vi "Read TopicLookupTable.vi"(11 "Mediator in":refnum<class "Mediator.lvclass">) -> (2 "TopicLookupTable":refnum<data-value>)   [LabVIEW 2018, in "MVA Framework.lvlib" / "Mediator.lvlib" / "Mediator.lvclass"]
doc: "读取主题查找表"
uses:
  Mediator.lvclass
  TopicLookupTable/TopicLookupTable.lvclass
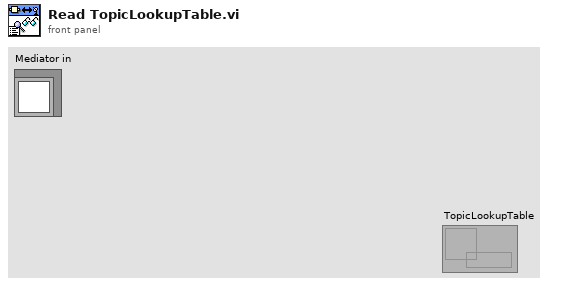
[diagram p1: front panel]
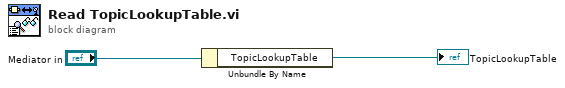
[diagram p0: block diagram]
diagram:
  n1 = Unbundle By Name("Mediator in") -> ("TopicLookupTable"=→"TopicLookupTable":refnum<data-value>)
